vi "COLORSENSORBUTTONCONTROL.vi"(2 "Spins":dbl, 3 "Spin?":bool) -> (0 "WOFMotorSpeed":dbl, 1 "Reset":bool)   [LabVIEW 2019]
uses:
  ArgosLib/Signal Processing/TypeDefs/EdgeDetector_Type.ctl
  ArgosLib/ArgosLib.lvlib
panel:
  in  "SpinTarget":dbl=3.5
  in  "Speed":dbl=1.0
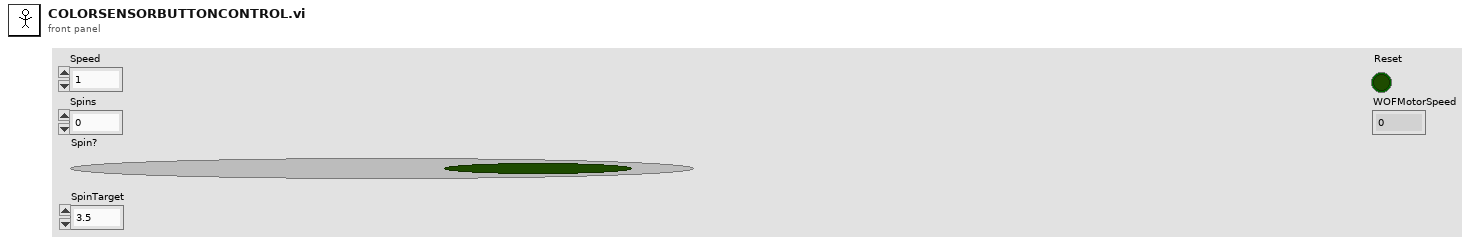
[diagram p1: front panel]
types:
  T1 = typedef "ArgosLib.lvlib/EdgeDetector_Type.ctl" = enum16{"RisingEdge", "FallingEdge", "Both"}
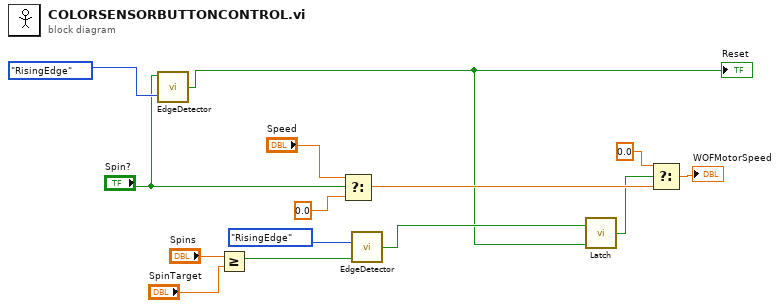
[diagram p0: block diagram]
diagram:
  n1 = call "EdgeDetector.vi"("DetectorType"=EdgeDetector_Type."RisingEdge", "Input"="Spin?") -> ("Edge"=w2:bool)
  "Reset" <- w2
  n2 = Greater Or Equal?(x="Spins", y="SpinTarget") -> (x >= y?=w10:bool)
  n3 = Select(t="Speed", s="Spin?", f=0.0) -> (s? t:f=w9:dbl)
  n4 = call "EdgeDetector.vi"("DetectorType"=EdgeDetector_Type."RisingEdge", "Input"=w10) -> ("Edge"=w3:bool)
  n5 = call "Latch.vi"("Reset"=w2, "Input"=w3) -> ("LatchOut"=w1:bool)
  n6 = Select(t=0.0, s=w1, f=w9) -> (s? t:f=→"WOFMotorSpeed":dbl)
